vi "RSZVB Get Fixed Frequency Signal Stage 2.vi"(8 "error in (no error)":errorcluster {"code" format="%.0x"}, 9 "Channel (1)":i32=1, 11 "VISA resource name":refnum<visa-resource-name>) -> (0 "error out":errorcluster {"code" format="%.0x"}, 2 "Fixed Frequency":i32, 3 "VISA resource name out":refnum<visa-resource-name>)   [LabVIEW 2011]
doc: "This VI returns the mixer input or output signal which is at the fixed frequency of second stage.\n\nRemote-control command(s):\n[SENSe<Ch>:]FREQuency:CONVersion:MIXer:FIXed2?"
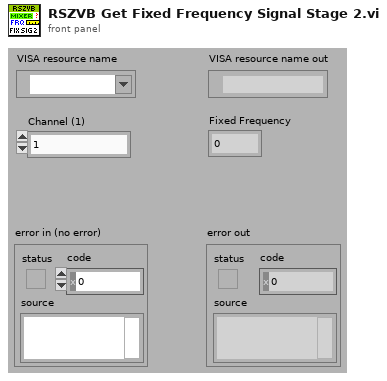
[diagram p1: front panel]
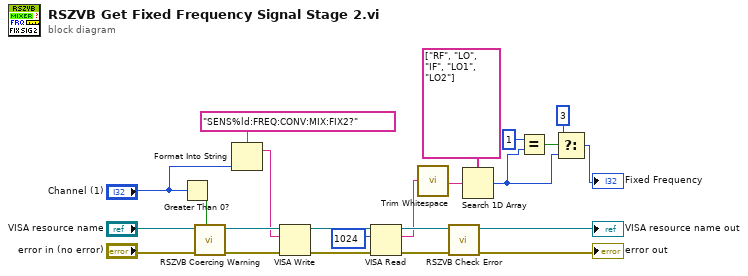
[diagram p0: block diagram]
diagram:
  n1 = Greater Than 0?(x="Channel (1)") -> (x > 0?=w14:bool)
  n2 = call "RSZVB Coercing Warning.vi"("In Range?"=w14, "error in (no error)"="error in (no error)", "VISA session"="VISA resource name") -> ("error out"=w21:errorcluster, "dup VISA session"=w22:refnum<visa-resource-name>)  [unwired: 7 in]
  n3 = Format Into String(format string="SENS%ld:FREQ:CONV:MIX:FIX2?", "Channel (1)") -> (resulting string=w20:string)  [unwired: 2 in, 1 out]
  n4 = VISA Write(VISA resource name=w22, write buffer=w20, error in (no error)=w21) -> (VISA resource name out=w17:refnum<visa-resource-name>, error out=w19:errorcluster)  [unwired: 1 out]
  n5 = VISA Read(VISA resource name=w17, byte count=u32 1024 ("byte count (0)"), error in (no error)=w19) -> (VISA resource name out=w16:refnum<visa-resource-name>, read buffer=w11:string, error out=w15:errorcluster)  [unwired: 1 out]
  n6 = call <vilib>:"Trim Whitespace.vi"("string"=w11) -> ("trimmed string"=w12:string)  [unwired: 1 in]
  n7 = call "RSZVB Check Error.vi"("error in (no error)"=w15, "VISA session"=w16) -> ("error out"=→"error out":errorcluster, "dup VISA session"=→"VISA resource name out":refnum<visa-resource-name>)  [unwired: 8 in]
  n8 = Search 1D Array(1D array=string[] ["RF", "LO", "IF", "LO1", "LO2"] ("array 2"), element=w12) -> (index of element=w2:i32)  [unwired: 1 in]
  n9 = Equal?(x=1, y=w2) -> (x = y?=w4:bool)
  n10 = Select(t=3, s=w4, f=w2) -> (s? t:f=→"Fixed Frequency":i32)
